vi "Day 10-1.vi"() -> ()   [LabVIEW 2019, in "Day 10.lvlib"]
uses:
  Day 10.lvlib
panel:
  out "Invalid":bool[](array[boolean])
  out "Corrupted":bool[](array[boolean])
  out "Array":i32[](array[numeric])
  out "Result":i32
  in  "String":string
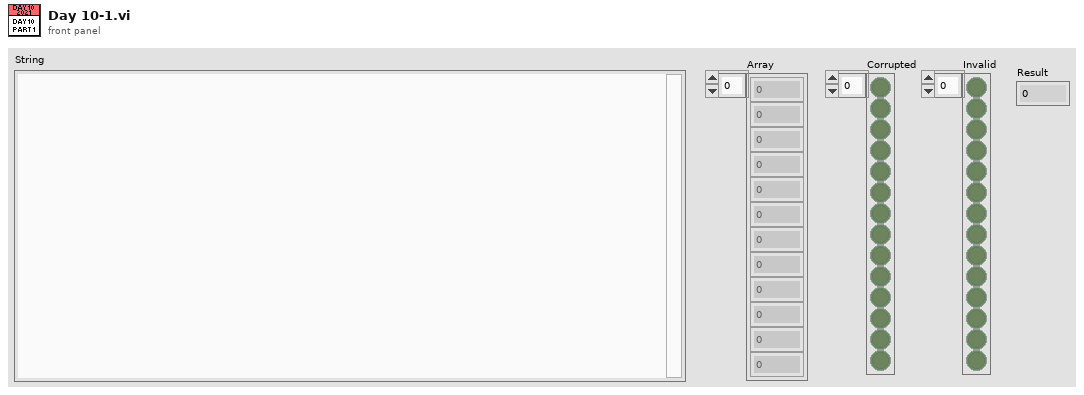
[diagram p1: front panel]
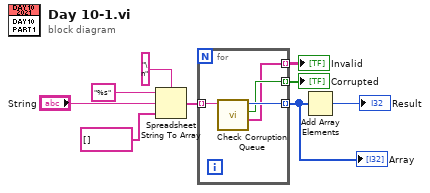
[diagram p0: block diagram]
diagram:
  n1 = Spreadsheet String To Array(delimiter (Tab)="\n", format string="%s", spreadsheet string="String", array type (2D Dbl)=string[] []) -> (array=w5:string[])
  n2 = for {
    tunnel: w5 -> [w13] mode=indexing
    tunnel: [w12] -> w4 mode=indexing
    tunnel: [w11] -> w2 mode=indexing
    tunnel: [w10] -> w1 mode=indexing
    n3 = call "Check Corruption Queue.vi"("input string"=w13) -> ("Remaining string"=w10:string[], "Corrupted?"=w11:bool, "Score"=w12:i32)  [unwired: 7 in, 1 out]
  }
  "Array" <- w4
  "Corrupted" <- w2
  "Invalid" <- w1
  n4 = Add Array Elements(numeric array=w4) -> (sum=→"Result":i32)
